vi "Swerve Drive.vi"(1 "Rot. Point Y":dbl, 3 "Rot. Point X":dbl, 12 "Auto Controls":bool=TRUE) -> ()   [LabVIEW 2016]
uses:
  Robot Global Data.vi
panel:
  in  "fr offset":dbl(knob)=178.773 scale=-180.0..180.0
  in  "fl offset":dbl(knob)=47.0 scale=-180.0..180.0
  in  "br offset":dbl(knob)=-138.0 scale=-180.0..180.0
  in  "bl offset":dbl(knob)=-144.0 scale=-180.0..180.0
  in  "Robot Length":dbl=21.2
  in  "Robot Width":dbl=20.125
  # "SWERVE DRIVE\nVersion 4.1\n\nApple Pi Robotics\nTeam 2067"
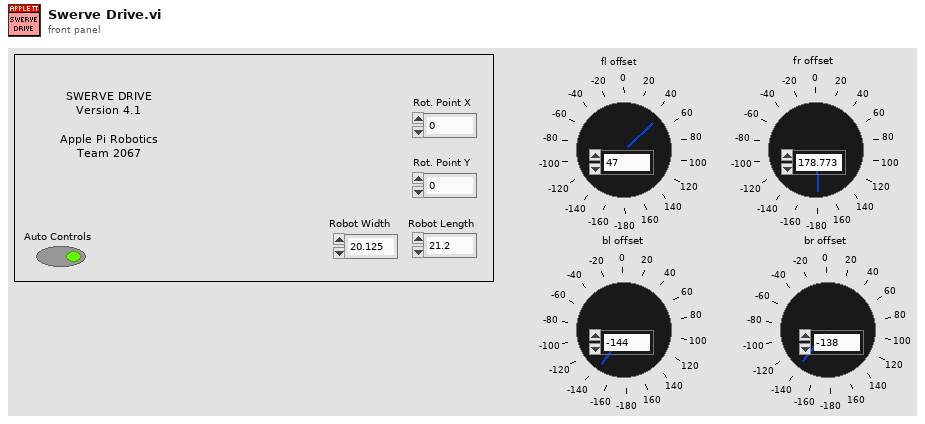
[diagram p1: front panel]
types:
  T1 = enum16{"Back Left", "Back Right", "Front Left", "Front Right"}
  T2 = typedef "WPI_MotorControlDeviceRef.ctl" = cluster{"DeviceStatus":errorcluster, "Type":T3, "PWM":cluster{"PWM Channel":T4, "DeadBand":T5}, "CAN":cluster{"Device Number":u8, "SetOutput VI Ref":variant, "GetOutput VI Ref":variant, "Enable VI Ref":variant, "Disable VI Ref":variant, "Data":variant}, "Invert":bool}
  T3 = typedef "WPI_MotorControlType.ctl" = enum16{"PWM", "CAN"}
  T4 = typedef "FPGA_DIOPWMChannel.ctl" = enum8{"PWM 0", "PWM 1", "PWM 2", "PWM 3", "PWM 4", "PWM 5", "PWM 6", "PWM 7", "PWM 8", "PWM 9", "PWM MXP 0", "PWM MXP 1", "PWM MXP 2", "PWM MXP 3", "PWM MXP 4", "PWM MXP 5", "PWM MXP 6", "PWM MXP 7", "PWM MXP 8", "PWM MXP 9", "Invalid"}
  T5 = typedef "WPI_PWMDeadband.ctl" = cluster{"Name":string, "maxPositivePwm":i32, "minPositivePwm":i32, "centerPwm":i32, "maxNegativePwm":i32, "minNegativePwm":i32, "angularRange":u16}
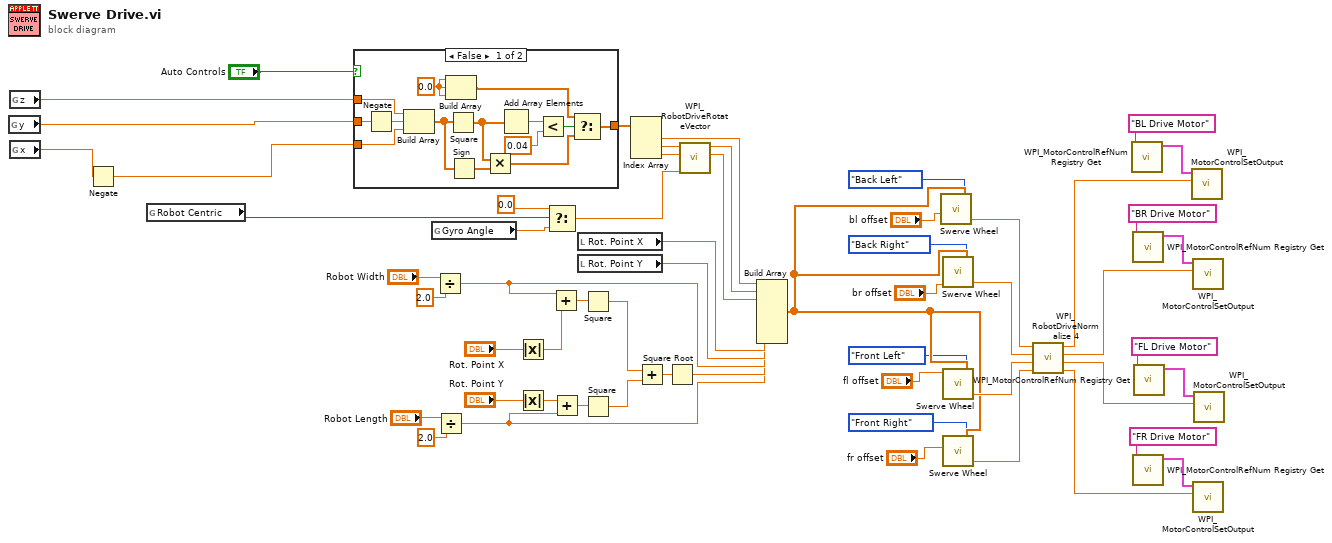
[diagram p0: block diagram]
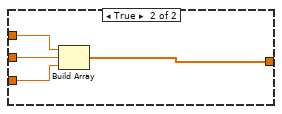
[diagram p2: hidden frame]
diagram:
  n1 = global read "Robot Global Data.vi" "y"() -> (w12:dbl)
  n2 = global read "Robot Global Data.vi" "z"() -> (w13:dbl)
  n3 = global read "Robot Global Data.vi" "x"() -> (w9:dbl)
  n4 = Negate(x=w9) -> (-x=w10:dbl)
  n5 = global read "Robot Global Data.vi" "Robot Centric"() -> (w11:bool)
  n6 = case shown="False" "Auto Controls" {
    tunnel: w12 -> [w69 w75]
    tunnel: w10 -> [w63 w76]
    tunnel: w13 -> [w59 w73]
    tunnel: [w60 w74] -> w22
    frame False {
      w67 = 0.0 ("element")
      n7 = Negate(x=w69) -> (-x=w62:dbl)
      n8 = Build Array(w59, w62, w63) -> (w66:dbl[])
      n9 = Build Array(w67, w67, w67) -> (w68:dbl[])
      n10 = Square(x=w66) -> (x^2=w64:dbl[])
      n11 = Sign(1:w66) -> (0:w65:dbl[])
      n12 = Multiply(x=w64, y=w65) -> (x*y=w61:dbl[])
      n13 = Add Array Elements(numeric array=w64) -> (sum=w72:dbl)
      n14 = Less?(x=w72, y=0.04 ("x")) -> (x < y?=w70:bool)
      n15 = Select(t=w68, s=w70, f=w61) -> (s? t:f=w60:dbl[])
    }
    frame True {
      n16 = Build Array(w73, w75, w76) -> (w74:dbl[])
    }
  }
  n17 = global read "Robot Global Data.vi" "Gyro Angle"() -> (w14:dbl)
  n18 = Divide(x="Robot Width", y=2.0) -> (x/y=w26:dbl)
  n19 = Divide(x="Robot Length", y=2.0) -> (x/y=w24:dbl)
  n20 = Absolute Value(x="Rot. Point X") -> (abs(x)=w42:dbl)
  n21 = Absolute Value(x="Rot. Point Y") -> (abs(x)=w40:dbl)
  n22 = Select(t=0.0, s=w11, f=w14) -> (s? t:f=w18:dbl)
  n23 = Add(x=w26, y=w42) -> (x+y=w41:dbl)
  n24 = Add(x=w40, y=w24) -> (x+y=w39:dbl)
  n25 = local read "Rot. Point X"() -> (w28:dbl)
  n26 = local read "Rot. Point Y"() -> (w27:dbl)
  n27 = Square(x=w41) -> (x^2=w37:dbl)
  n28 = Square(x=w39) -> (x^2=w38:dbl)
  n29 = Index Array(array=w22) -> (element #1=w17:dbl, element #2=w23:dbl, element #3=w29:dbl)  [unwired: 3 in]
  n30 = Add(x=w37, y=w38) -> (x+y=w36:dbl)
  n31 = Square Root(x=w36) -> (sqrt(x)=w25:dbl)
  n32 = call <vilib>:"WPI_RobotDriveRotateVector.vi"("Angle"=w18, "X"=w29, "Y"=w23) -> ("X'"=w20:dbl, "Y'"=w16:dbl)  [unwired: 7 out]
  n33 = Build Array(w17, w16, w20, w28, w27, w26, w25, w24) -> (w21:dbl[])
  n34 = call "Swerve Wheel.vi"("Wheel"=T1."Back Left", "Inputs"=w21, "bl offset"="bl offset") -> ("Speed"=w58:dbl)  [unwired: 3 in]
  n35 = call "Swerve Wheel.vi"("Wheel"=T1."Back Right", "Inputs"=w21, "br offset"="br offset") -> ("Speed"=w57:dbl)  [unwired: 3 in]
  n36 = call "Swerve Wheel.vi"("Wheel"=T1."Front Left", "Inputs"=w21, "fl offset"="fl offset") -> ("Speed"=w56:dbl)  [unwired: 3 in]
  n37 = call "Swerve Wheel.vi"("Wheel"=T1."Front Right", "Inputs"=w21, "fr offset"="fr offset") -> ("Speed"=w55:dbl)  [unwired: 3 in]
  n38 = call <vilib>:"WPI_RobotDriveNormalize 4.vi"("D"=w55, "C"=w56, "B"=w57, "A"=w58) -> ("D'"=w43:dbl, "C'"=w44:dbl, "B'"=w45:dbl, "A'"=w46:dbl)
  n39 = call <vilib>:"WPI_MotorControlRefNum Registry Get.vi"("refnum name"="BL Drive Motor") -> ("MotorControlDevRef"=w54:T2)  [unwired: 9 in, 1 out]
  n40 = call <vilib>:"WPI_MotorControlRefNum Registry Get.vi"("refnum name"="BR Drive Motor") -> ("MotorControlDevRef"=w51:T2)  [unwired: 9 in, 1 out]
  n41 = call <vilib>:"WPI_MotorControlRefNum Registry Get.vi"("refnum name"="FR Drive Motor") -> ("MotorControlDevRef"=w47:T2)  [unwired: 9 in, 1 out]
  n42 = call <vilib>:"WPI_MotorControlRefNum Registry Get.vi"("refnum name"="FL Drive Motor") -> ("MotorControlDevRef"=w50:T2)  [unwired: 9 in, 1 out]
  n43 = call <vilib>:"WPI_MotorControlSetOutput.vi"("Output"=w46, "MotorControlDevRef"=w54) -> ()  [unwired: 7 in, 3 out]
  n44 = call <vilib>:"WPI_MotorControlSetOutput.vi"("Output"=w45, "MotorControlDevRef"=w51) -> ()  [unwired: 7 in, 3 out]
  n45 = call <vilib>:"WPI_MotorControlSetOutput.vi"("Output"=w43, "MotorControlDevRef"=w47) -> ()  [unwired: 7 in, 3 out]
  n46 = call <vilib>:"WPI_MotorControlSetOutput.vi"("Output"=w44, "MotorControlDevRef"=w50) -> ()  [unwired: 7 in, 3 out]
